vi "useOneROIFindRectangel.vi"(0 "Image Dst In":T4, 1 "Edge Polarity Array":T2[](array[typedef])=[{"Edge Polarity"=0, "Kernel Size"=3, "Width"=3, "Minimum Edge Strength"=10.0, "Interpolation Type"=enum."Bilinear Fixed", "Data Processing Method"=enum."Average"}, {"Edge Polarity"=0, "Kernel Size"=3, "Width"=3, "Minimum Edge Strength"=10.0, "Interpolation Type"=enum."Bilinear Fixed", "Data Processing Method"=enum."Average"}, {"Edge Polarity"=0, "Kernel Size"=3, "Width"=3, "Minimum Edge Strength"=10.0, "Interpolation Type"=enum."Bilinear Fixed", "Data Processing Method"=enum."Average"}, {"Edge Polarity"=0, "Kernel Size"=3, "Width"=3, "Minimum Edge Strength"=10.0, "Interpolation Type"=enum."Bilinear Fixed", "Data Processing Method"=enum."Average"}] {"Edge Polarity" items=["All Edges", "Rising Edges", "Falling Edges"]; "Minimum Edge Strength" format="%.2f"; "Width" step=2; "Kernel Size" step=2}, 5 "ROI Descriptor":T5 {"Contours"."Type" items=["No Selection", "Point", "Line", "Rectangle", "Oval", "Polygon", "Freehand Region", "Annulus", "Unused2", "Unused3", "Broken Line", "Freehand Line", "Rotated Rectangle"]}, 7 "SearchArea(0.3)":dbl=0.3 format="%#_13g", 9 "Options":T1={"Show Search Area"=FALSE, "Show Search Lines"=FALSE, "Show Edges Found"=FALSE, "Show Result"=TRUE, "Search Area Color"=16711680, "Search Lines Color"=255, "Edge Locations Color"=16776960, "Result Color"=64255, "Overlay Group Name"="", "Show Search Area 2"=FALSE, "Show Search Lines 2"=FALSE, "Show Edges Found 2"=FALSE, "Show Result 2"=TRUE, "Search Area Color 2"=16711680, "Search Lines Color 2"=255, "Edge Locations Color 2"=16776960, "Result Color 2"=16744448, "Overlay Group Name 2"="", "Show Search Area 3"=FALSE, "Show Search Lines 3"=FALSE, "Show Edges Found 3"=FALSE, "Show Result 3"=TRUE, "Search Area Color 3"=16711680, "Search Lines Color 3"=255, "Edge Locations Color 3"=16776960, "Result Color 3"=16776960, "Overlay Group Name 3"="", "Show Search Area 4"=FALSE, "Show Search Lines 4"=FALSE, "Show Edges Found 4"=FALSE, "Show Result 4"=TRUE, "Search Area Color 4"=16711680, "Search Lines Color 4"=255, "Edge Locations Color 4"=16776960, "Result Color 4"=64000, "Overlay Group Name 4"="", "Show 4 Edge Point Result"=TRUE, "Show 4 Edge Result "=TRUE, " 4 Edge Point Result Color "=16711680, " 4 Edge Result Color "=255}, 11 "error In":errorcluster) -> (4 "Image Dst Out":T4, 15 "error Out":errorcluster)   [LabVIEW 2015]
uses:
  <vilib>/vision/Image Controls.llb/IMAQ Image.ctl
  <vilib>/vision/Measure.llb/Edge Options.ctl
  <vilib>/vision/Measure.llb/Edge Polarity.ctl
  <vilib>/vision/NI_Vision_Development_Module.lvlib
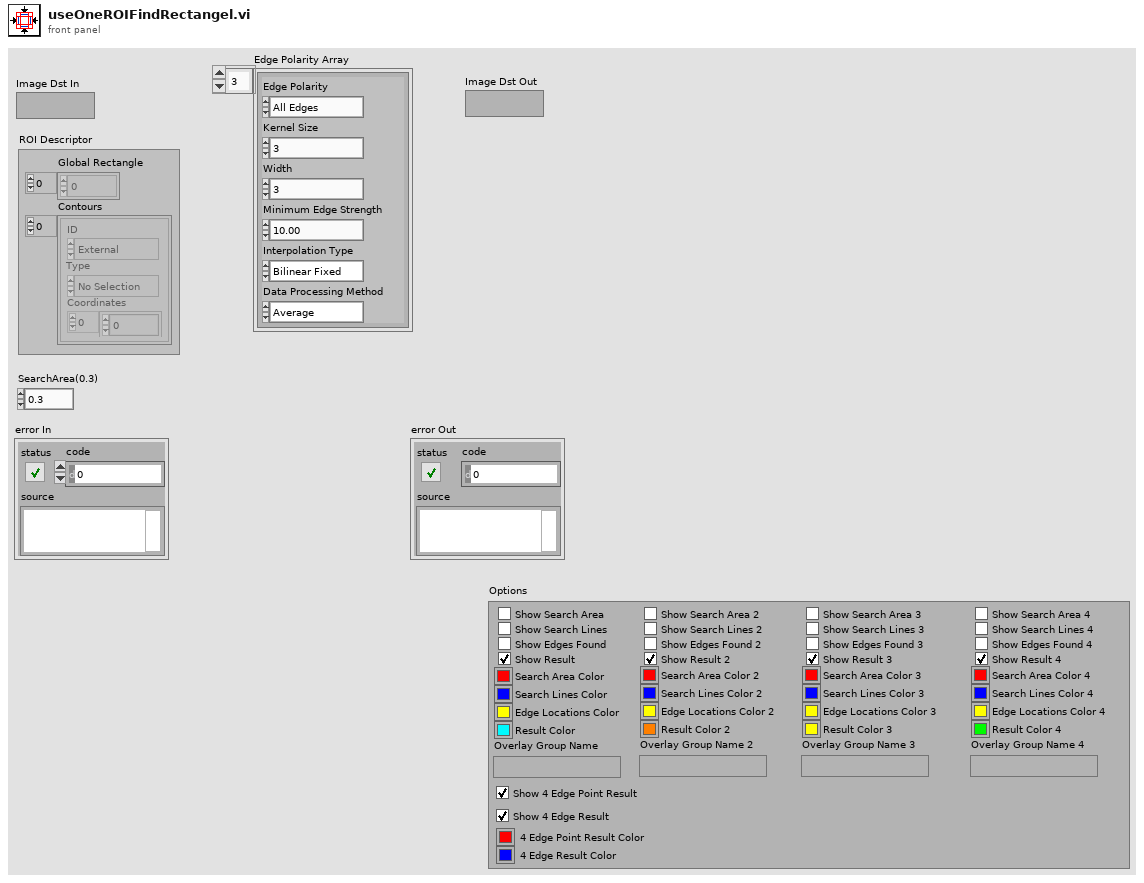
[diagram p1: front panel]
types:
  T1 = cluster{"Show Search Area":bool, "Show Search Lines":bool, "Show Edges Found":bool, "Show Result":bool, "Search Area Color":u32, "Search Lines Color":u32, "Edge Locations Color":u32, "Result Color":u32, "Overlay Group Name":string, "Show Search Area 2":bool, "Show Search Lines 2":bool, "Show Edges Found 2":bool, "Show Result 2":bool, "Search Area Color 2":u32, "Search Lines Color 2":u32, "Edge Locations Color 2":u32, "Result Color 2":u32, "Overlay Group Name 2":string, "Show Search Area 3":bool, "Show Search Lines 3":bool, "Show Edges Found 3":bool, "Show Result 3":bool, "Search Area Color 3":u32, "Search Lines Color 3":u32, "Edge Locations Color 3":u32, "Result Color 3":u32, "Overlay Group Name 3":string, "Show Search Area 4":bool, "Show Search Lines 4":bool, "Show Edges Found 4":bool, "Show Result 4":bool, "Search Area Color 4":u32, "Search Lines Color 4":u32, "Edge Locations Color 4":u32, "Result Color 4":u32, "Overlay Group Name 4":string, "Show 4 Edge Point Result":bool, "Show 4 Edge Result ":bool, " 4 Edge Point Result Color ":u32, " 4 Edge Result Color ":u32}
  T2 = typedef "Edge Options.ctl" = cluster{"Edge Polarity":T3, "Kernel Size":u32, "Width":u32, "Minimum Edge Strength":sgl, "Interpolation Type":enum32{"Zero Order", "Bilinear", "Quadratic", "Cubic", "Bilinear Fixed"}, "Data Processing Method":enum32{"Average", "Median"}}
  T3 = typedef "Edge Polarity.ctl" = u32
  T4 = typedef "IMAQ Image.ctl" = refnum<image>
  T5 = typedef "ROI Descriptor" = cluster{"Global Rectangle":i32[], "Contours":cluster{"ID":enum32{"External", "Internal"}, "Type":u32, "Coordinates":i32[]}[]}
  T6 = cluster{"Left":i32, "Top":i32, "Right":i32, "Bottom":i32}
  T7 = cluster{"Global Rectangle":i32[], "Contours":cluster{"ID":enum32{"External", "Internal"}, "Type":u32, "Coordinates":i32[]}[]}
  T8 = cluster{"Point 1":cluster{"X":sgl, "Y":sgl}, "Point 2":cluster{"X":sgl, "Y":sgl}}
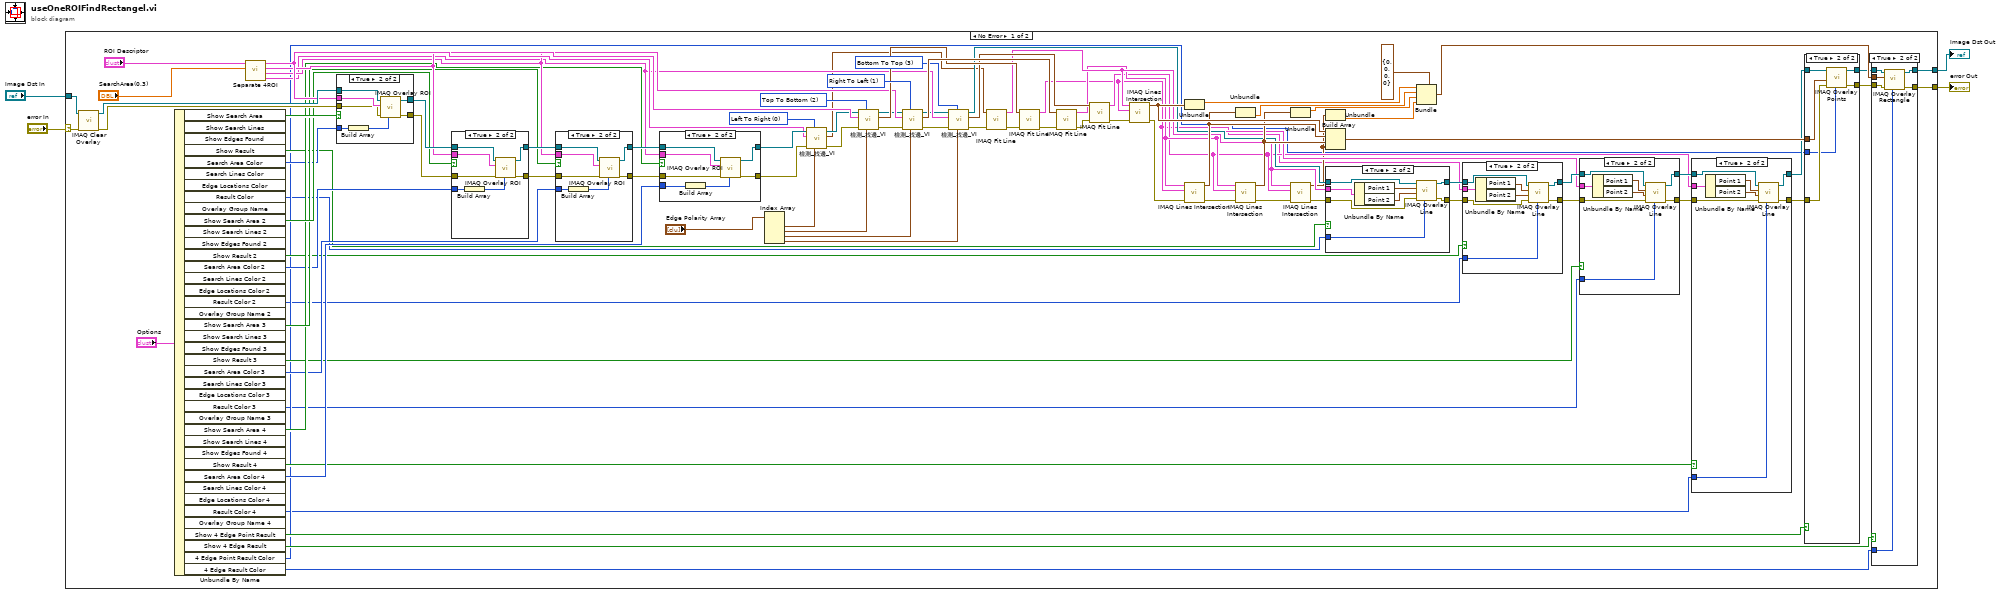
[diagram p0: block diagram]
diagram:
  n1 = case shown="No Error" "error In" {
    selector: "error In" -> [w74 w192]
    tunnel: "Image Dst In" -> [w99 w193]
    tunnel: [w63 w193] -> w2
    tunnel: [w61 w192] -> w1
    frame No Error {
      w93 = u16 2 items=["Left To Right", "Right To Left", "Top To Bottom", "Bottom To Top"] ("Scan Direction")
      w51 = u16 3 items=["Left To Right", "Right To Left", "Top To Bottom", "Bottom To Top"] ("Scan Direction")
      w97 = u16 1 items=["Left To Right", "Right To Left", "Top To Bottom", "Bottom To Top"] ("Scan Direction")
      w98 = u16 0 items=["Left To Right", "Right To Left", "Top To Bottom", "Bottom To Top"] ("Scan Direction")
      n2 = call "IMAQ Clear Overlay"("error in (no error)"=w74, "Image"=w99) -> ("error out"=w75:errorcluster, "Image Out"=w86:T4)  [unwired: 8 in]
      n3 = Unbundle By Name("Options") -> ("Show Search Area"=w24:bool, "Show Result"=w16:bool, "Search Area Color"=w20:u32, "Result Color"=w8:u32, "Show Search Area 2"=w23:bool, "Show Result 2"=w15:bool, "Search Area Color 2"=w19:u32, "Result Color 2"=w6:u32, "Show Search Area 3"=w22:bool, "Show Result 3"=w14:bool, "Search Area Color 3"=w18:u32, "Result Color 3"=w5:u32, "Show Search Area 4"=w21:bool, "Show Result 4"=w13:bool, "Search Area Color 4"=w17:u32, "Result Color 4"=w7:u32, "Show 4 Edge Point Result"=w11:bool, "Show 4 Edge Result"=w12:bool, "4 Edge Point Result Color"=w10:u32, "4 Edge Result Color"=w9:u32)  [unwired: 20 out]
      n4 = call "Separate 4ROI.vi"("SearchArea(0.5)"="SearchArea(0.3)", "ROI Descriptor"="ROI Descriptor") -> ("Bottom ROI"=w78:T7, "Right ROI"=w79:T7, "Top ROI"=w80:T7, "Left ROI"=w81:T7)  [unwired: 2 in]
      n5 = case shown="True" w24 {
        tunnel: [w183 w191] -> w87
        tunnel: w86 -> [w184 w190]
        tunnel: [w184 w189] -> w85
        tunnel: w81 -> [_ w188]
        tunnel: w75 -> [w183 w187]
        tunnel: w20 -> [_ w185]
        frame False {
        }
        frame True {
          n6 = Build Array(w185) -> (w186:u32[])
          n7 = call "IMAQ Overlay ROI"("Colors (Green)"=w186, "error in (no error)"=w187, "ROI Descriptor"=w188, "Image"=w190) -> ("error out"=w191:errorcluster, "Image Out"=w189:T4)  [unwired: 6 in]
        }
      }
      n8 = case shown="True" w23 {
        tunnel: w87 -> [w174 w182]
        tunnel: w85 -> [w175 w181]
        tunnel: [w175 w180] -> w84
        tunnel: w80 -> [_ w179]
        tunnel: [w174 w178] -> w58
        tunnel: w19 -> [_ w176]
        frame False {
        }
        frame True {
          n9 = Build Array(w176) -> (w177:u32[])
          n10 = call "IMAQ Overlay ROI"("Colors (Green)"=w177, "error in (no error)"=w182, "ROI Descriptor"=w179, "Image"=w181) -> ("error out"=w178:errorcluster, "Image Out"=w180:T4)  [unwired: 6 in]
        }
      }
      n11 = case shown="True" w22 {
        tunnel: w84 -> [w166 w173]
        tunnel: [w166 w172] -> w83
        tunnel: w79 -> [_ w171]
        tunnel: w58 -> [w165 w170]
        tunnel: [w165 w169] -> w57
        tunnel: w18 -> [_ w167]
        frame False {
        }
        frame True {
          n12 = Build Array(w167) -> (w168:u32[])
          n13 = call "IMAQ Overlay ROI"("Colors (Green)"=w168, "error in (no error)"=w170, "ROI Descriptor"=w171, "Image"=w173) -> ("error out"=w169:errorcluster, "Image Out"=w172:T4)  [unwired: 6 in]
        }
      }
      n14 = case shown="True" w21 {
        tunnel: w83 -> [w157 w164]
        tunnel: [w157 w163] -> w82
        tunnel: w78 -> [_ w162]
        tunnel: w57 -> [w156 w161]
        tunnel: [w156 w160] -> w50
        tunnel: w17 -> [_ w158]
        frame False {
        }
        frame True {
          n15 = Build Array(w158) -> (w159:u32[])
          n16 = call "IMAQ Overlay ROI"("Colors (Green)"=w159, "error in (no error)"=w161, "ROI Descriptor"=w162, "Image"=w164) -> ("error out"=w160:errorcluster, "Image Out"=w163:T4)  [unwired: 6 in]
        }
      }
      n17 = Index Array(array="Edge Polarity Array") -> (element #1=w59:T2, element #2=w39:T2, element #3=w38:T2, element #4=w37:T2)  [unwired: 4 in]
      n18 = call "檢測_找邊_VI.vi"("Edge Options"=w59, "Scan Direction"=w98, "error in (no error)"=w50, "ROI"=w81, "Image"=w82) -> ("error out"=w49:errorcluster, "Array"=w43:cluster{"X":sgl, "Y":sgl}[], "Image Out"=w48:T4)  [unwired: 4 in]
      n19 = call "檢測_找邊_VI.vi"("Edge Options"=w39, "Scan Direction"=w93, "error in (no error)"=w49, "ROI"=w80, "Image"=w48) -> ("error out"=w45:errorcluster, "Array"=w94:cluster{"X":sgl, "Y":sgl}[], "Image Out"=w47:T4)  [unwired: 4 in]
      n20 = call "檢測_找邊_VI.vi"("Edge Options"=w38, "Scan Direction"=w97, "error in (no error)"=w45, "ROI"=w79, "Image"=w47) -> ("error out"=w44:errorcluster, "Array"=w96:cluster{"X":sgl, "Y":sgl}[], "Image Out"=w46:T4)  [unwired: 4 in]
      n21 = call "檢測_找邊_VI.vi"("Edge Options"=w37, "Scan Direction"=w51, "error in (no error)"=w44, "ROI"=w78, "Image"=w46) -> ("error out"=w92:errorcluster, "Array"=w52:cluster{"X":sgl, "Y":sgl}[], "Image Out"=w56:T4)  [unwired: 4 in]
      n22 = call "IMAQ Fit Line"("error in (no error)"=w92, "Points"=w43) -> ("error out"=w42:errorcluster, "Line Segment"=w30:T8)  [unwired: 4 in, 4 out]
      n23 = call "IMAQ Fit Line"("error in (no error)"=w42, "Points"=w94) -> ("error out"=w41:errorcluster, "Line Segment"=w26:T8)  [unwired: 4 in, 4 out]
      n24 = call "IMAQ Fit Line"("error in (no error)"=w41, "Points"=w96) -> ("error out"=w40:errorcluster, "Line Segment"=w29:T8)  [unwired: 4 in, 4 out]
      n25 = call "IMAQ Fit Line"("error in (no error)"=w40, "Points"=w52) -> ("error out"=w91:errorcluster, "Line Segment"=w28:T8)  [unwired: 4 in, 4 out]
      n26 = call "IMAQ Lines Intersection"("error in (no error)"=w91, "Line 2"=w26, "Line 1"=w30) -> ("error out"=w90:errorcluster, "Intersection Point"=w73:cluster{"X":sgl, "Y":sgl})  [unwired: 6 in, 1 out]
      n27 = Unbundle(w73) -> ("X"=w70:sgl)  [unwired: 1 out]
      n28 = call "IMAQ Lines Intersection"("error in (no error)"=w90, "Line 2"=w26, "Line 1"=w29) -> ("error out"=w89:errorcluster, "Intersection Point"=w72:cluster{"X":sgl, "Y":sgl})  [unwired: 6 in, 1 out]
      n29 = Unbundle(w72) -> ("Y"=w69:sgl)  [unwired: 1 out]
      n30 = call "IMAQ Lines Intersection"("error in (no error)"=w89, "Line 2"=w28, "Line 1"=w29) -> ("error out"=w88:errorcluster, "Intersection Point"=w71:cluster{"X":sgl, "Y":sgl})  [unwired: 6 in, 1 out]
      n31 = Unbundle(w71) -> ("X"=w68:sgl)  [unwired: 1 out]
      n32 = call "IMAQ Lines Intersection"("error in (no error)"=w88, "Line 2"=w28, "Line 1"=w30) -> ("error out"=w54:errorcluster, "Intersection Point"=w27:cluster{"X":sgl, "Y":sgl})  [unwired: 6 in, 1 out]
      n33 = Unbundle(w27) -> ("Y"=w67:sgl)  [unwired: 1 out]
      n34 = Build Array(w73, w72, w71, w27) -> (w95:cluster{"X":sgl, "Y":sgl}[])
      n35 = case shown="True" w16 {
        tunnel: w56 -> [w147 w153]
        tunnel: [w147 w152] -> w36
        tunnel: w8 -> [_ w151]
        tunnel: w54 -> [w146 w150]
        tunnel: [w146 w149] -> w33
        tunnel: w30 -> [_ w148]
        frame False {
        }
        frame True {
          n36 = Unbundle By Name(w148) -> ("Point 1"=w155:cluster{"X":sgl, "Y":sgl}, "Point 2"=w154:cluster{"X":sgl, "Y":sgl})
          n37 = call "IMAQ Overlay Line"("Color"=w151, "error in (no error)"=w150, "End Point"=w154, "Start Point"=w155, "Image"=w153) -> ("error out"=w149:errorcluster, "Image Out"=w152:T4)  [unwired: 5 in]
        }
      }
      n38 = Bundle(cluster=T6 {"Left"=0, "Top"=0, "Right"=0, "Bottom"=0} ("Rectangle"), "Left"=w70, "Top"=w69, "Right"=w68, "Bottom"=w67) -> (w65:T6)
      n39 = case shown="True" w15 {
        tunnel: w26 -> [_ w135]
        tunnel: w36 -> [w127 w132]
        tunnel: [w127 w131] -> w35
        tunnel: w6 -> [_ w130]
        tunnel: w33 -> [w126 w129]
        tunnel: [w126 w128] -> w32
        frame False {
        }
        frame True {
          n40 = Unbundle By Name(w135) -> ("Point 1"=w134:cluster{"X":sgl, "Y":sgl}, "Point 2"=w133:cluster{"X":sgl, "Y":sgl})
          n41 = call "IMAQ Overlay Line"("Color"=w130, "error in (no error)"=w129, "End Point"=w133, "Start Point"=w134, "Image"=w132) -> ("error out"=w128:errorcluster, "Image Out"=w131:T4)  [unwired: 5 in]
        }
      }
      n42 = case shown="True" w14 {
        tunnel: w29 -> [_ w145]
        tunnel: w35 -> [w137 w142]
        tunnel: [w137 w141] -> w34
        tunnel: w5 -> [_ w140]
        tunnel: w32 -> [w136 w139]
        tunnel: [w136 w138] -> w31
        frame False {
        }
        frame True {
          n43 = Unbundle By Name(w145) -> ("Point 1"=w144:cluster{"X":sgl, "Y":sgl}, "Point 2"=w143:cluster{"X":sgl, "Y":sgl})
          n44 = call "IMAQ Overlay Line"("Color"=w140, "error in (no error)"=w139, "End Point"=w143, "Start Point"=w144, "Image"=w142) -> ("error out"=w138:errorcluster, "Image Out"=w141:T4)  [unwired: 5 in]
        }
      }
      n45 = case shown="True" w13 {
        tunnel: w28 -> [_ w125]
        tunnel: w34 -> [w117 w122]
        tunnel: [w117 w121] -> w55
        tunnel: w7 -> [_ w120]
        tunnel: w31 -> [w116 w119]
        tunnel: [w116 w118] -> w53
        frame False {
        }
        frame True {
          n46 = Unbundle By Name(w125) -> ("Point 1"=w124:cluster{"X":sgl, "Y":sgl}, "Point 2"=w123:cluster{"X":sgl, "Y":sgl})
          n47 = call "IMAQ Overlay Line"("Color"=w120, "error in (no error)"=w119, "End Point"=w123, "Start Point"=w124, "Image"=w122) -> ("error out"=w118:errorcluster, "Image Out"=w121:T4)  [unwired: 5 in]
        }
      }
      n48 = case shown="True" w11 {
        tunnel: w95 -> [_ w107]
        tunnel: [w100 w106] -> w64
        tunnel: [w101 w105] -> w62
        tunnel: w55 -> [w100 w104]
        tunnel: w53 -> [w101 w103]
        tunnel: w10 -> [_ w102]
        frame False {
        }
        frame True {
          n49 = call "IMAQ Overlay Points"("Color"=w102, "error in (no error)"=w103, "Array of Points"=w107, "Image"=w104) -> ("error out"=w105:errorcluster, "Image Out"=w106:T4)  [unwired: 6 in]
        }
      }
      n50 = case shown="True" w12 {
        tunnel: w65 -> [_ w115]
        tunnel: w64 -> [w109 w114]
        tunnel: [w109 w113] -> w63
        tunnel: w62 -> [w108 w112]
        tunnel: [w108 w111] -> w61
        tunnel: w9 -> [_ w110]
        frame False {
        }
        frame True {
          n51 = call "IMAQ Overlay Rectangle"("Color"=w110, "error in (no error)"=w112, "Rectangle"=w115, "Image"=w114) -> ("error out"=w111:errorcluster, "Image Out"=w113:T4)  [unwired: 6 in]
        }
      }
    }
    frame Error {
    }
  }
  "Image Dst Out" <- w2
  "error Out" <- w1
